vi "Get Status Register.vi"(8 "error in (no error)":errorcluster, 10 "Board no.":i32, 11 "TDCManager":T1) -> (0 "error out":errorcluster, 2 "Status register":i64, 3 "TDCManager":T1)   [LabVIEW 2016, in "HPTDC Driver Library.lvlib"]
uses:
  HPTDC Driver Library.lvlib
  Typedefs/TDCManager.ctl
  C:/Users/CRT Controller/CRTC Labview Application/Source/HPTDC Driver Library Folder/Library files/hptdc_net4_3.7.0_x64.dll
  hptdc_net4_3.7.0_x64.dll
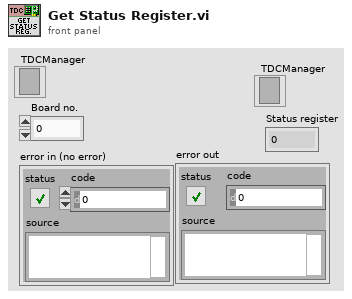
[diagram p1: front panel]
types:
  T1 = typedef "HPTDC Driver Library.lvlib/TDCManager.ctl" = refnum<k24>
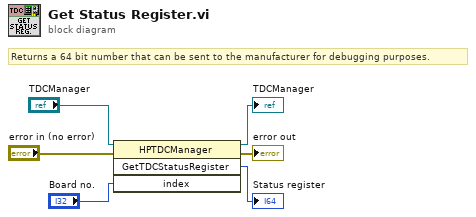
[diagram p0: block diagram]
diagram:
  # "Returns a 64 bit number that can be sent to the manufacturer for debugging purposes."
  n1 = invoke class="HPTDCManager" method="GetTDCStatusRegister"(reference="TDCManager", error in="error in (no error)", "index"="Board no.") -> (reference out=→"TDCManager":T1, error out=→"error out":errorcluster, "GetTDCStatusRegister"=→"Status register":i64)  [unwired: 1 in, 1 out]
